vi "Find Click Zone Wheel Index.vi"(7 "picture info":T3={"picture size"={"Width"=500, "Height"=500}, "pixels per unit"=10.0}, 8 "error in (no error)":errorcluster, 9 "pixel tolerance (5)":i32=5, 10 "picture coordinate":cluster{"x":i32, "y":i32}, 11 "click zones group":T2) -> (0 "error out":errorcluster, 1 "found?":bool, 2 "wheel index":i32, 4 "global mouse position":cluster{"x":dbl, "y":dbl})   [LabVIEW 2017, in "NI_Robotics_Configure Steering Frame.lvlib"]
uses:
  <vilib>/robotics/Dialog/Configure Steering Frame/NI_Robotics_Configure Steering Frame.lvlib
  <vilib>/robotics/Utilities/Visualization/Steering Visualization/Steering Picture/Picture Info.ctl
  <vilib>/Utility/miscctls.llb/LVBoundsTypeDef.ctl
  <vilib>/robotics/Dialog/Configure Steering Frame/Click Zone.ctl
  <vilib>/robotics/Utilities/Visualization/Steering Visualization/Steering Picture/NI_Robotics_Steering Picture.lvlib
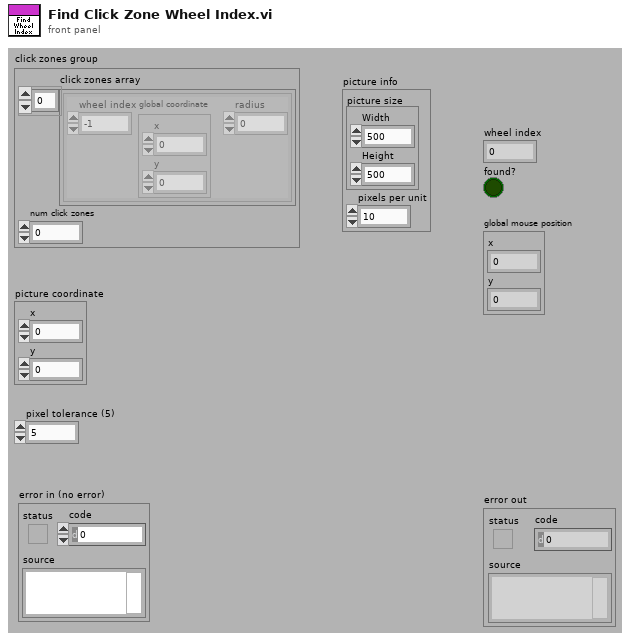
[diagram p1: front panel]
types:
  T1 = typedef "NI_Robotics_Configure Steering Frame.lvlib/Click Zone.ctl" = cluster{"wheel index":i32, "global coordinate":cluster{"x":dbl, "y":dbl}, "radius":dbl}
  T2 = cluster{"click zones array":T1[], "num click zones":i32}
  T3 = typedef "NI_Robotics_Steering Picture.lvlib/Picture Info.ctl" = cluster{"picture size":T4, "pixels per unit":dbl}
  T4 = typedef "LVBoundsTypeDef.ctl" = cluster{"Width":u32, "Height":u32}
  T5 = cluster{"elements":T1[], "number of elements":i32}
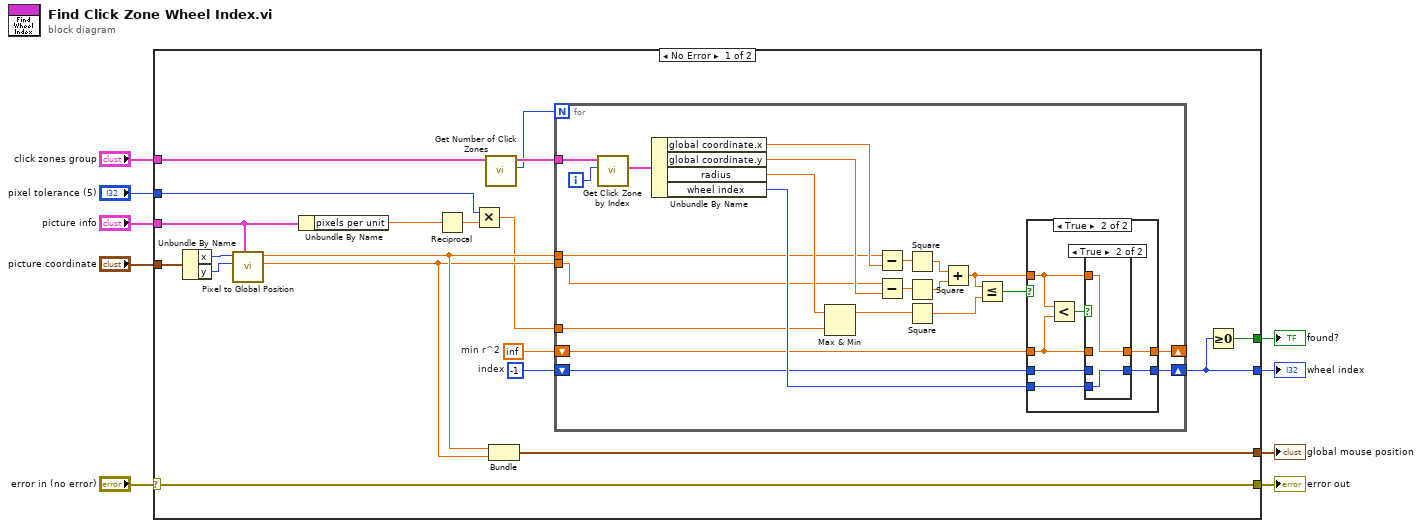
[diagram p0: block diagram]
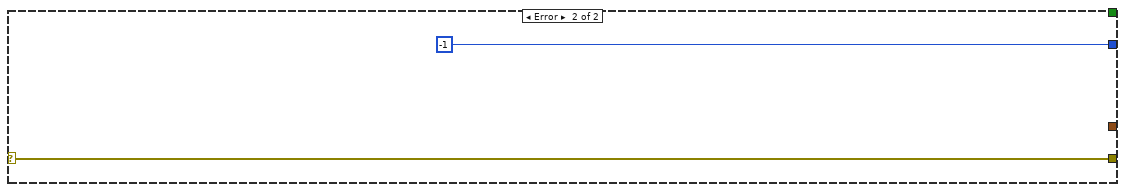
[diagram p4: hidden frame]
diagram:
  n1 = case shown="No Error" "error in (no error)" {
    selector: "error in (no error)" -> [w13 w65]
    tunnel: "picture coordinate" -> [w24 _]
    tunnel: "picture info" -> [w23 _]
    tunnel: "pixel tolerance (5)" -> [w22 _]
    tunnel: "click zones group" -> [w21 _]
    tunnel: [w13 w65] -> w4
    tunnel: [w12 _] -> w3
    tunnel: [w11 -1 ("index")] -> w2
    tunnel: [w10 _] -> w1
    frame No Error {
      w17 = -1  # index
      w18 = inf  # min r^2
      n2 = Unbundle By Name(w24) -> ("x"=w25:i32, "y"=w26:i32)
      n3 = call <vilib>:"Pixel to Global Position.vi"("picture info"=w23, "pixel y"=w26, "pixel x"=w25) -> ("global y"=w15:dbl, "global x"=w16:dbl)  [unwired: 7 in]
      n4 = Unbundle By Name(w23) -> ("pixels per unit"=w27:dbl)
      n5 = Reciprocal(x=w27) -> (1/x=w28:dbl)
      n6 = Multiply(x=w22, y=w28) -> (x*y=w14:dbl)
      n7 = call <vilib>:"Get Number of Click Zones.vi"("array in"=w21) -> ("number of click zones"=w19:i32, "array out"=w20:T5)  [unwired: 9 in]
      n8 = Bundle("global x"=w16, "global y"=w15) -> (w12:cluster{"global x":dbl, "global y":dbl})  [unwired: 1 in]
      n9 = for {
        N: w19 -> [_]
        tunnel: w20 -> [w50]
        shift-right: [w30] -> _
        shift-left: w18 -> [w32]
        shift-right: [w29] -> w11
        shift-left: w17 -> [w31]
        tunnel: w16 -> [w35]
        tunnel: w15 -> [w34]
        tunnel: w14 -> [w33]
        i -> [w49]
        n10 = call <vilib>:"Get Click Zone by Index.vi"("index"=w49, "array in"=w50) -> ("click zone"=w36:T1)  [unwired: 7 in, 2 out]
        n11 = Unbundle By Name(w36) -> ("global coordinate.x"=w37:dbl, "global coordinate.y"=w38:dbl, "radius"=w47:dbl, "wheel index"=w44:i32)
        n12 = Max & Min(x=w47, y=w33) -> (max(x,y)=w48:dbl)  [unwired: 1 out]
        n13 = Subtract(x=w35, y=w37) -> (x-y=w45:dbl)
        n14 = Subtract(x=w34, y=w38) -> (x-y=w46:dbl)
        n15 = Square(x=w45) -> (x^2=w40:dbl)
        n16 = Square(x=w46) -> (x^2=w39:dbl)
        n17 = Square(x=w48) -> (x^2=w41:dbl)
        n18 = Add(x=w40, y=w39) -> (x+y=w43:dbl)
        n19 = Less Or Equal?(x=w43, y=w41) -> (x <= y?=w42:bool)
        n20 = case shown="True" w42 {
          tunnel: w43 -> [_ w59]
          tunnel: w32 -> [w52 w58]
          tunnel: [w52 w55] -> w30
          tunnel: w31 -> [w51 w57]
          tunnel: [w51 w54] -> w29
          tunnel: w44 -> [_ w56]
          frame False {
          }
          frame True {
            n21 = Less?(x=w59, y=w58) -> (x < y?=w53:bool)
            n22 = case shown="True" w53 {
              tunnel: w59 -> [_ w63]
              tunnel: w58 -> [w61 _]
              tunnel: w57 -> [w60 _]
              tunnel: w56 -> [_ w62]
              tunnel: [w61 w63] -> w55
              tunnel: [w60 w62] -> w54
              frame False {
              }
              frame True {
              }
            }
          }
        }
      }
      n23 = Greater Or Equal To 0?(x=w11) -> (x >= 0?=w10:bool)
    }
    frame Error {
    }
  }
  "error out" <- w4
  "wheel index" <- w2
  "found?" <- w1
  "global mouse position" <- w3
